vi "S2C_XML_CreateAsset.vi"(8 "Error In":errorcluster, 11 "AssetData":T1) -> (0 "Error Out":errorcluster)   [LabVIEW 2015]
uses:
  S2C_XML_Globals.vi
  <vilib>/xml/Close Reference(Node).vi
  <resource>/objmgr/DOMUserDefRef.rc
  <vilib>/xml/NI_XML.lvlib
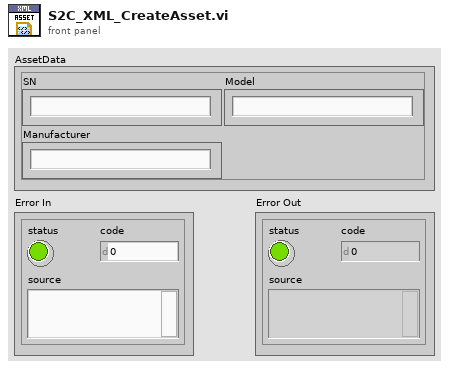
[diagram p1: front panel]
types:
  T1 = cluster{"SN":string, "Manufacturer":string, "Model":string}
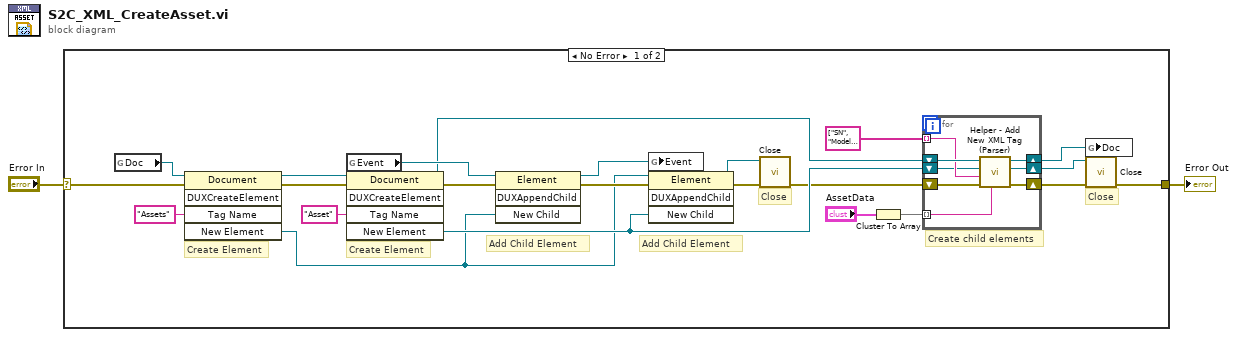
[diagram p0: block diagram]
diagram:
  n1 = case shown="No Error" "Error In" {
    selector: "Error In" -> [w24 w34]
    tunnel: [w3 w34] -> w2
    frame No Error {
      # "Close"
      # "Close"
      # "Create child elements"
      # "Add Child Element"
      # "Create Element"
      # "Add Child Element"
      # "Create Element"
      n2 = global read "S2C_XML_Globals.vi" "Doc"() -> (w18:refnum<k20>)
      n3 = invoke class="Document" method="DUXCreateElement"(reference=w18, error in=w24, "Tag Name"="Assets") -> (reference out=w23:refnum<k20>, error out=w22:errorcluster, "New Element"=w7:refnum<k20>)  [unwired: 2 in, 2 out]
      n4 = global read "S2C_XML_Globals.vi" "Event"() -> (w17:refnum<k20>)
      n5 = invoke class="Document" method="DUXCreateElement"(reference=w23, error in=w22, "Tag Name"="Asset") -> (reference out=w14:refnum<k20>, error out=w19:errorcluster, "New Element"=w13:refnum<k20>)  [unwired: 2 in, 2 out]
      n6 = invoke class="Element" method="DUXAppendChild"(reference=w17, error in=w19, "New Child"=w7) -> (reference out=w8:refnum<k20>, error out=w20:errorcluster)  [unwired: 1 in, 2 out]
      n7 = global write "S2C_XML_Globals.vi" "Event"(w8) -> ()
      n8 = invoke class="Element" method="DUXAppendChild"(reference=w7, error in=w20, "New Child"=w13) -> (reference out=w5:refnum<k20>, error out=w6:errorcluster)  [unwired: 1 in, 2 out]
      n9 = call-poly <vilib>:"Close.vi"("error in (no error)"=w6, "node"=w5) -> ("error out"=w4:errorcluster)  [unwired: 7 in]
      n10 = Cluster To Array(cluster="AssetData") -> (array=w16:string[])
      n11 = for {
        tunnel: w16 -> [w31] mode=indexing
        tunnel: string[] ["SN", "Model", "Manufacturer"] -> [w30] mode=indexing
        shift-right: [w29] -> w10
        shift-left: w14 -> [w33]
        shift-right: [w27] -> w11
        shift-left: w4 -> [w32]
        shift-right: [w26] -> w9
        shift-left: w13 -> [w28]
        n12 = call "Helper - Add New XML Tag (Parser).vi"("Tag Data"=w31, "error in (no error)"=w32, "Tag Name"=w30, "Owning Element"=w28, "DOM document"=w33) -> ("error out"=w27:errorcluster, "dup Owning Element"=w26:refnum<k20>, "dup DOM document"=w29:refnum<k20>)  [unwired: 4 in]
      }
      n13 = global write "S2C_XML_Globals.vi" "Doc"(w10) -> ()
      n14 = call-poly <vilib>:"Close.vi"("error in (no error)"=w11, "node"=w9) -> ("error out"=w3:errorcluster)  [unwired: 7 in]
    }
    frame Error {
    }
  }
  "Error Out" <- w2
